vi "Set Table Row Active.vi"(1 "Current Step ID":i32, 2 "Test Table":refnum<vi>) -> ()   [LabVIEW 2018]
uses:
  <vilib>/Utility/miscctls.llb/LVRowAndColumnTypeDef.ctl
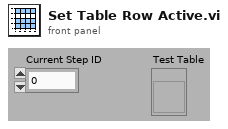
[diagram p1: front panel]
types:
  T1 = typedef "LVRowAndColumnTypeDef.ctl" = cluster{"Row":i32, "Column":i32}
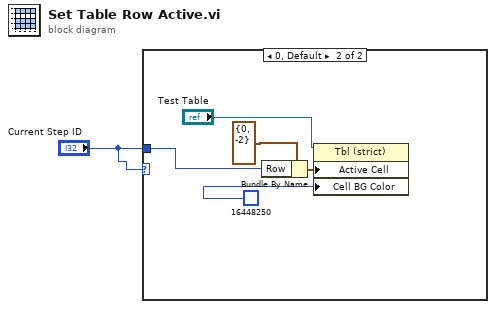
[diagram p0: block diagram]
diagram:
  n1 = case shown="0, Default" "Current Step ID" {
    tunnel: "Current Step ID" -> [_ w5]
    frame ..-1 {
    }
    frame 0, Default {
      n2 = Bundle By Name(cluster=T1 {"Row"=0, "Column"=-2} ("Active Cell:Active Cell"), "Row"=w5) -> (w3:T1)
      n3 = property class="Tbl (strict)"(reference="Test Table", "Active Cell"=w3, "Cell BG Color"=u32 16448250 ("Color Box")) -> ()  [unwired: 1 in, 2 out]
    }
  }
